vi "Golander pump(mL per s, mL per rev).vi"(4 "State":i16, 5 "Time":dbl format="%.2f", 6 "Sensor Values":dbl[](array[numeric]), 7 "Set Points":dbl[](array[numeric])) -> (0 "required data":T4={"Set Point names"=["com port", "pump address", "pump (mL/rev)", "flow (mL/s)"], "required number of setpoints"=4, "required number of sensors"=0, "Sensor names"=[]}, 3 "output value":dbl)   [LabVIEW 2015]
uses:
  modbusrtu/MB Serial Master Query Write Single Register (poly).vi
  modbusrtu/MB Serial Master Query Read Holding Registers (poly).vi
panel:
  out "pump cmd array":T1(array[cluster])
  out "output cluster":T2
  in  "cluster":T3
  in  "error in (no error)":errorcluster
  out "VISA out":refnum<visa-resource-name>
  out "error out":errorcluster
  # "Enter the correct information for this control code in the required data structure below. Then make the current value default by right clicking on the border of the data structure. Select \"data operations\" and then select \"make current value default\". These values will be displayed by process controller."
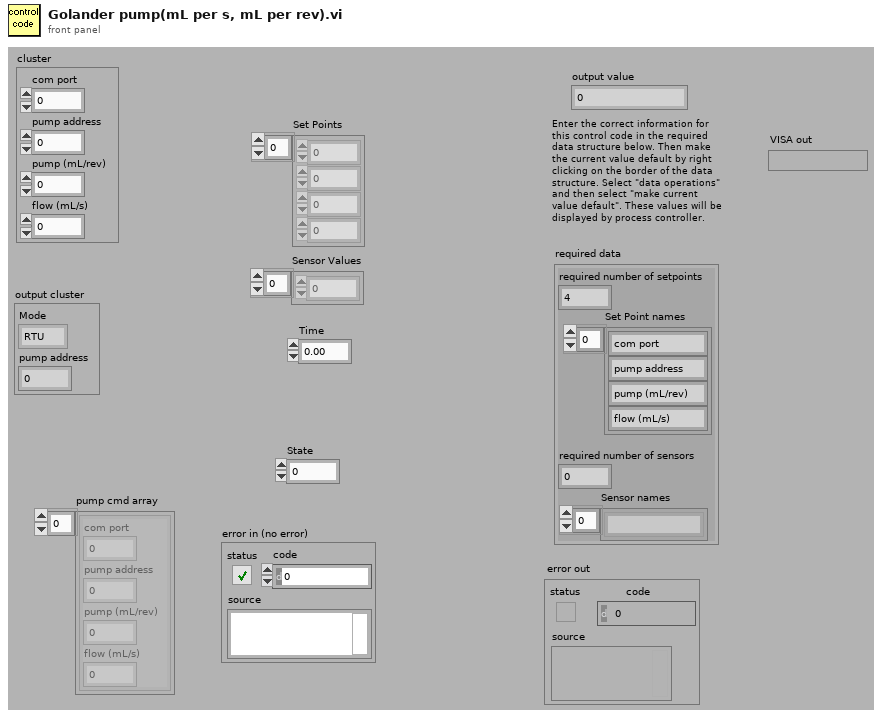
[diagram p1: front panel]
types:
  T1 = cluster{"com port":u8, "pump address":u8, "pump (mL/rev)":dbl, "flow (mL/s)":dbl}[]
  T2 = cluster{"Mode":enum16{"RTU", "ASCII"}, "pump address":u8}
  T3 = cluster{"com port":u8, "pump address":u8, "pump (mL/rev)":dbl, "flow (mL/s)":dbl}
  T4 = cluster{"Set Point names":string[], "required number of setpoints":u8, "required number of sensors":u8, "Sensor names":string[]}
  T5 = cluster{"Set Points[0]":dbl, "Set Points[1]":dbl, "Set Points[2]":dbl, "Set Points[3]":dbl}
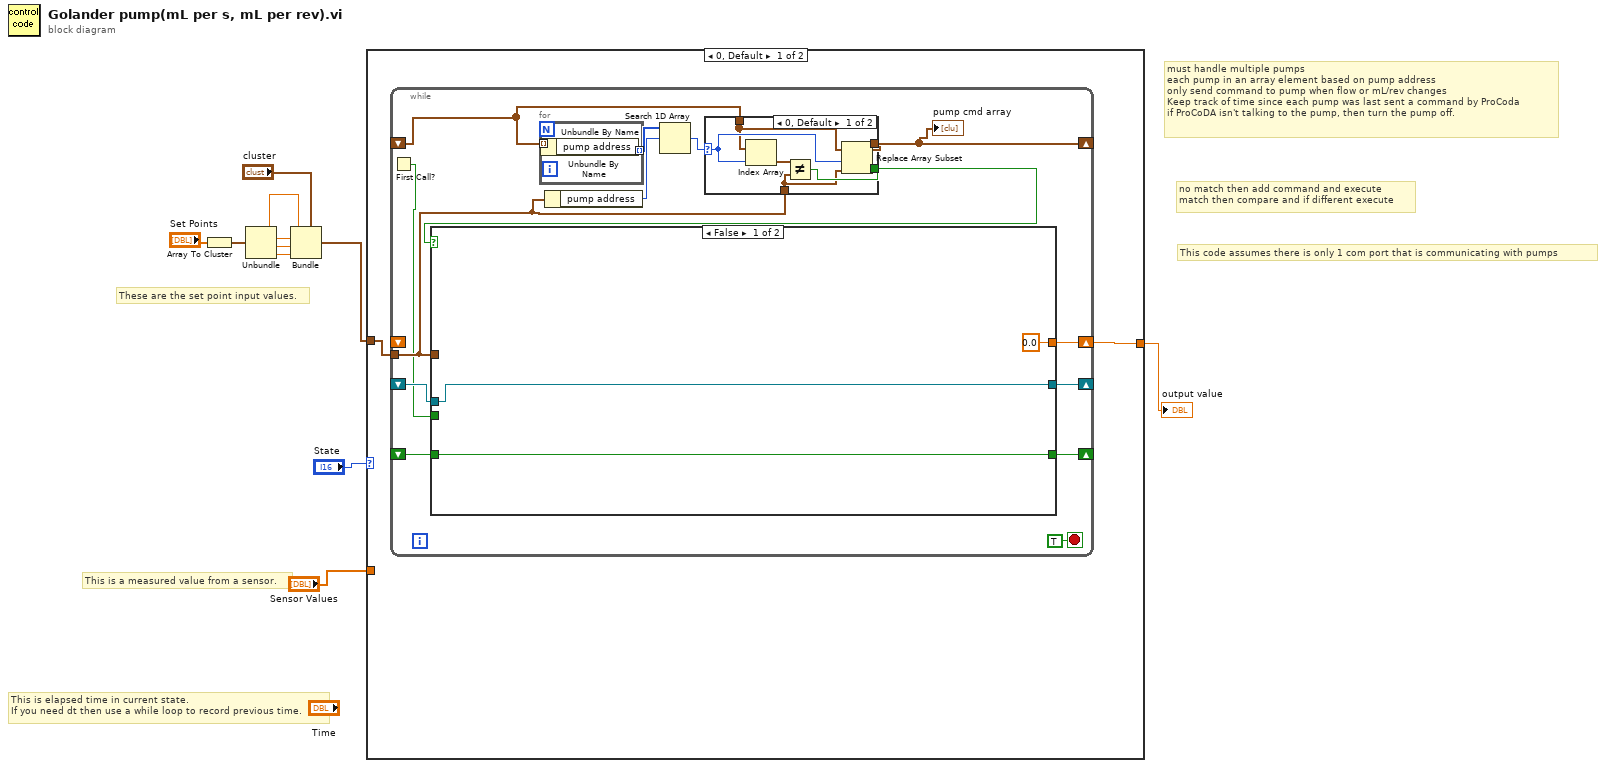
[diagram p0: block diagram]
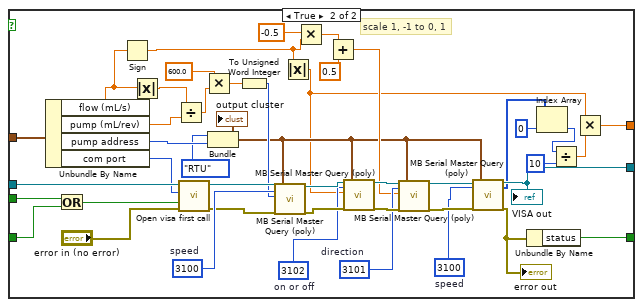
[diagram p2: hidden frame]
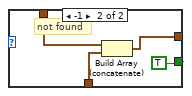
[diagram p3: hidden frame]
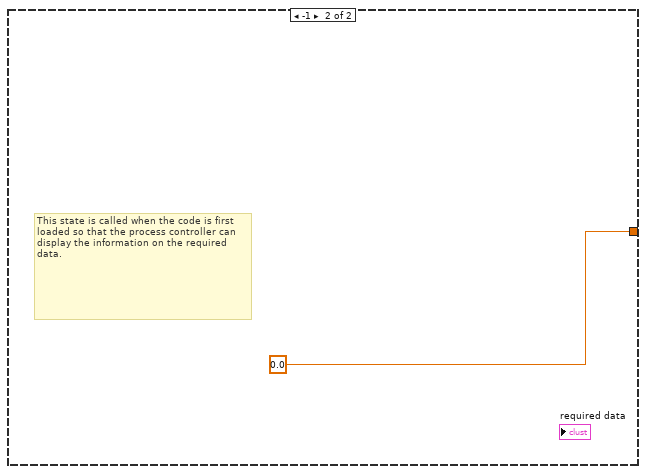
[diagram p4: hidden frame]
diagram:
  # "This code assumes there is only 1 com port that is communicating with pumps"
  # "no match then add command and execute\nmatch then compare and if different execute"
  # "must handle multiple pumps\neach pump in an array element based on pump address\nonly send command to pump when flow or mL/rev changes\nKeep track of time since each pump was last sent a command by ProCoda\nif ProCoDA isn't talking to the pump, then turn the pump off."
  # "These are the set point input values."
  # "This is a measured value from a sensor."
  # "This is elapsed time in current state.\nIf you need dt then use a while loop to record previous time."
  n1 = Array To Cluster(array="Set Points") -> (cluster=w8:T5)
  n2 = Unbundle(w8) -> ("Set Points[0]"=w4:dbl, "Set Points[1]"=w9:dbl, "Set Points[2]"=w3:dbl, "Set Points[3]"=w2:dbl)
  n3 = Bundle(cluster="cluster", "com port"=w4, "pump address"=w9, "pump (mL/rev)"=w3, "flow (mL/s)"=w2) -> (w6:T3)
  n4 = case shown="0, Default" "State" {
    tunnel: [w12 0.0 ("fraction on")] -> w1
    tunnel: w6 -> [w13 _]
    tunnel: "Sensor Values" -> [_ _]
    frame 0, Default {
      n5 = while {
        shift-right: [w23] -> _
        shift-left: _ -> [w26]
        tunnel: w13 -> [w17]
        shift-right: [w24] -> _
        shift-left: _ -> [w25]
        shift-right: [w15] -> _
        shift-left: _ -> [w14]
        shift-right: [w22] -> w12
        shift-left: _ -> [_]
        stop <- TRUE stop-if-true
        n6 = First Call?() -> (First Call?: T/F=w16:bool)
        n7 = for {
          tunnel: [w86] -> w21 mode=indexing
          tunnel: w14 -> [w85] mode=indexing
          n8 = Unbundle By Name(w85) -> ("pump address"=w86:u8)
        }
        n9 = Unbundle By Name(w17) -> ("pump address"=w20:u8)
        n10 = Search 1D Array(1D array=w21, element=w20) -> (index of element=w19:i32)  [unwired: 1 in]
        n11 = case shown="0, Default" w19 {
          selector: w19 -> [w77 _]
          tunnel: [w79 TRUE] -> w18
          tunnel: w14 -> [w76 w83]
          tunnel: w17 -> [w78 w82]
          tunnel: [w75 w81] -> w15
          frame 0, Default {
            n12 = Index Array(array=w76, index=w77) -> (element=w80:T3)
            n13 = Not Equal?(x=w80, y=w78) -> (x != y?=w79:bool)
            n14 = Replace Array Subset(array=w76, new element=w78, index=w77) -> (w75:T1)
          }
          frame -1 {
            # "not found"
            n15 = Build Array (concatenate)(w83, w82) -> (w81:T1)
          }
        }
        "pump cmd array" <- w15
        n16 = case shown="False" w18 {
          tunnel: w26 -> [w30 w73]
          tunnel: w25 -> [w29 w71]
          tunnel: [w29 w70] -> w24
          tunnel: [w30 w45] -> w23
          tunnel: [0.0 w34] -> w22
          tunnel: w17 -> [_ w32]
          tunnel: w16 -> [_ w31]
          frame False {
          }
          frame True {
            w42 = u16 3100  # speed
            w51 = u16 3101  # direction
            w54 = u16 3102  # on or off
            w60 = u16 3100  # speed
            # "scale 1, -1 to 0, 1"
            n17 = Unbundle By Name(w32) -> ("flow (mL/s)"=w61:dbl, "pump (mL/rev)"=w65:dbl, "pump address"=w67:u8, "com port"=w69:u8)
            n18 = Or(x=w31, y=w71) -> (x .or. y?=w72:bool)
            n19 = Sign(1:w61) -> (0:w50:dbl)
            n20 = Absolute Value(x=w61) -> (abs(x)=w62:dbl)
            n21 = Divide(x=w62, y=w65) -> (x/y=w64:dbl)
            n22 = call "Open visa first call.vi"("error in (no error)"="error in (no error)", "First Call?: T/F"=w72, "Com port"=w69, "VISA Refnum in"=w73) -> ("error out"=w57:errorcluster, "VISA Refnum out"=w68:refnum<visa-resource-name>)  [unwired: 6 in]
            n23 = Multiply(x=600.0, y=w64) -> (x*y=w59:dbl)
            n24 = Bundle("Mode"=enum16{"RTU", "ASCII"}."RTU", "pump address"=w67) -> (w41:T2)  [unwired: 1 in]
            "output cluster" <- w41
            n25 = To Unsigned Word Integer(number=w59) -> (unsigned 16bit integer=w58:u16)
            n26 = call-poly "MB Serial Master Query (poly).vi"("VISA resource name"=w68, "Address"=w60, "Holding Register"=w58, "error in"=w57, "Serial Parameters"=w41) -> ("VISA resource name out"=w55:refnum<visa-resource-name>, "error out"=w56:errorcluster)  [unwired: 12 in, 1 out]
            n27 = Absolute Value(x=w50) -> (abs(x)=w36:dbl)
            n28 = Multiply(x=-0.5, y=w50) -> (x*y=w48:dbl)
            n29 = Add(x=w48, y=0.5) -> (x+y=w46:dbl)
            n30 = call-poly "MB Serial Master Query (poly).vi"("VISA resource name"=w55, "Address"=w54, "Holding Register"=w36, "error in"=w56, "Serial Parameters"=w41) -> ("VISA resource name out"=w53:refnum<visa-resource-name>, "error out"=w52:errorcluster)  [unwired: 12 in, 1 out]
            n31 = call-poly "MB Serial Master Query (poly).vi"("VISA resource name"=w53, "Address"=w51, "Holding Register"=w46, "error in"=w52, "Serial Parameters"=w41) -> ("VISA resource name out"=w43:refnum<visa-resource-name>, "error out"=w44:errorcluster)  [unwired: 12 in, 1 out]
            n32 = call-poly "MB Serial Master Query (poly).vi"("VISA resource name"=w43, "Starting Address"=w42, "error in"=w44, "Serial Parameters"=w41) -> ("VISA resource name out"=w45:refnum<visa-resource-name>, "Holding Registers"=w39:u16[], "error out"=w33:errorcluster)  [unwired: 12 in, 1 out]
            "VISA out" <- w45
            "error out" <- w33
            n33 = Unbundle By Name(w33) -> ("status"=w70:bool)
            n34 = Index Array(array=w39, index=0) -> (element=w38:u16)
            n35 = Divide(x=w38, y=u16 10) -> (x/y=w35:dbl)
            n36 = Multiply(x=w36, y=w35) -> (x*y=w34:dbl)
          }
        }
      }
    }
    frame -1 {
      # "This state is called when the code is first loaded so that the process controller can display the information on the required data."
    }
  }
  "output value" <- w1
